vi "ColorScale.vi"(4 "Width":i32=100, 6 "Height":i32=450, 8 "ColorMap":T1=59 items=["Bathymetry9", "BlackBody", "Blue", "BlueBlackRed", "BlueGreenOrange", "BlueHot", "BlueHot256", "BlueRedGreen", "BlueRedGreen256", "BrownViolet", "Classification", "ColdWarm", "Copper", "Cyan", "CyanMagenta", "Cycles", "dBZ14", "dBZ21", "EOSOrangeBlue11", "EOSSpectral11", "Fiddle", "Geo", "Geo32", "Gold", "Grays", "Grays16", "Grays256", "Green", "GreenMagenta16", "LandAndSea", "LandAndSea8", "Magenta", "Mocha", "Mud", "Pastels", "PastelsMap", "PastelsMap20", "PlanetEarth", "PlanetEarth256", "Rainbow", "Rainbow4Cycles", "Rainbow16", "Rainbow256", "RainbowCycle", "Red", "RedWhiteBlue", "RedWhiteBlue256", "RedWhiteGreen", "Relief", "Relief19", "SeaLandAndFire", "Spectrum", "SpectrumBlack", "Terrain", "Terrain256", "VioletOrangeYellow", "Web216", "Yellow", "YellowHot", "YellowHot256"], 9 "Low":i32, 10 "High":i32=260) -> (3 "ColorScale":picture)   [LabVIEW 2014]
uses:
  <vilib>/picture/picture.llb/Draw True-Color Pixmap.vi
  ColorMaps.ctl
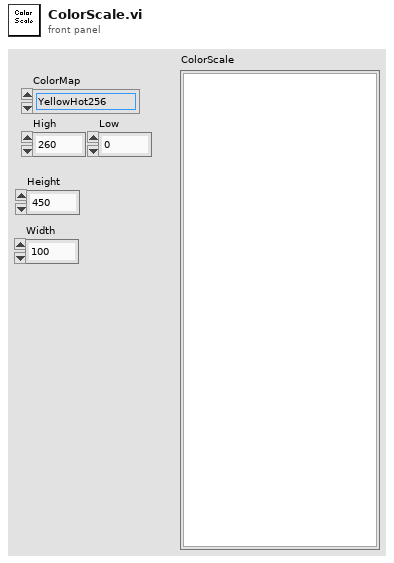
[diagram p1: front panel]
types:
  T1 = typedef "ColorMaps.ctl" = u16
  T2 = cluster{"Width":i16, "Style":enum32{"Solid", "Dash", "Dot", "DashDot", "DashDotDot"}}
  T3 = cluster{"left":i16, "top":i16, "right":i16, "bottom":i16}
  T4 = cluster{"format":enum8{"Decimal", "Scientific", "Engineering", "Binary", "Octal", "Hex"}, "precision":u8}
  T5 = cluster{"horizontal":bool, "left/top":bool, "draw bar":bool, "line color":u32, "text color(black)":u32}
  T6 = cluster{"coordinate 1":i16, "value 1":dbl, "coordinate 2":i16, "value 2":dbl, "log?(F)":bool, "fmt and prec":cluster{"format":enum8{"Decimal", "Scientific", "Engineering", "Binary", "Octal", "Hex"}, "precision":u8}}
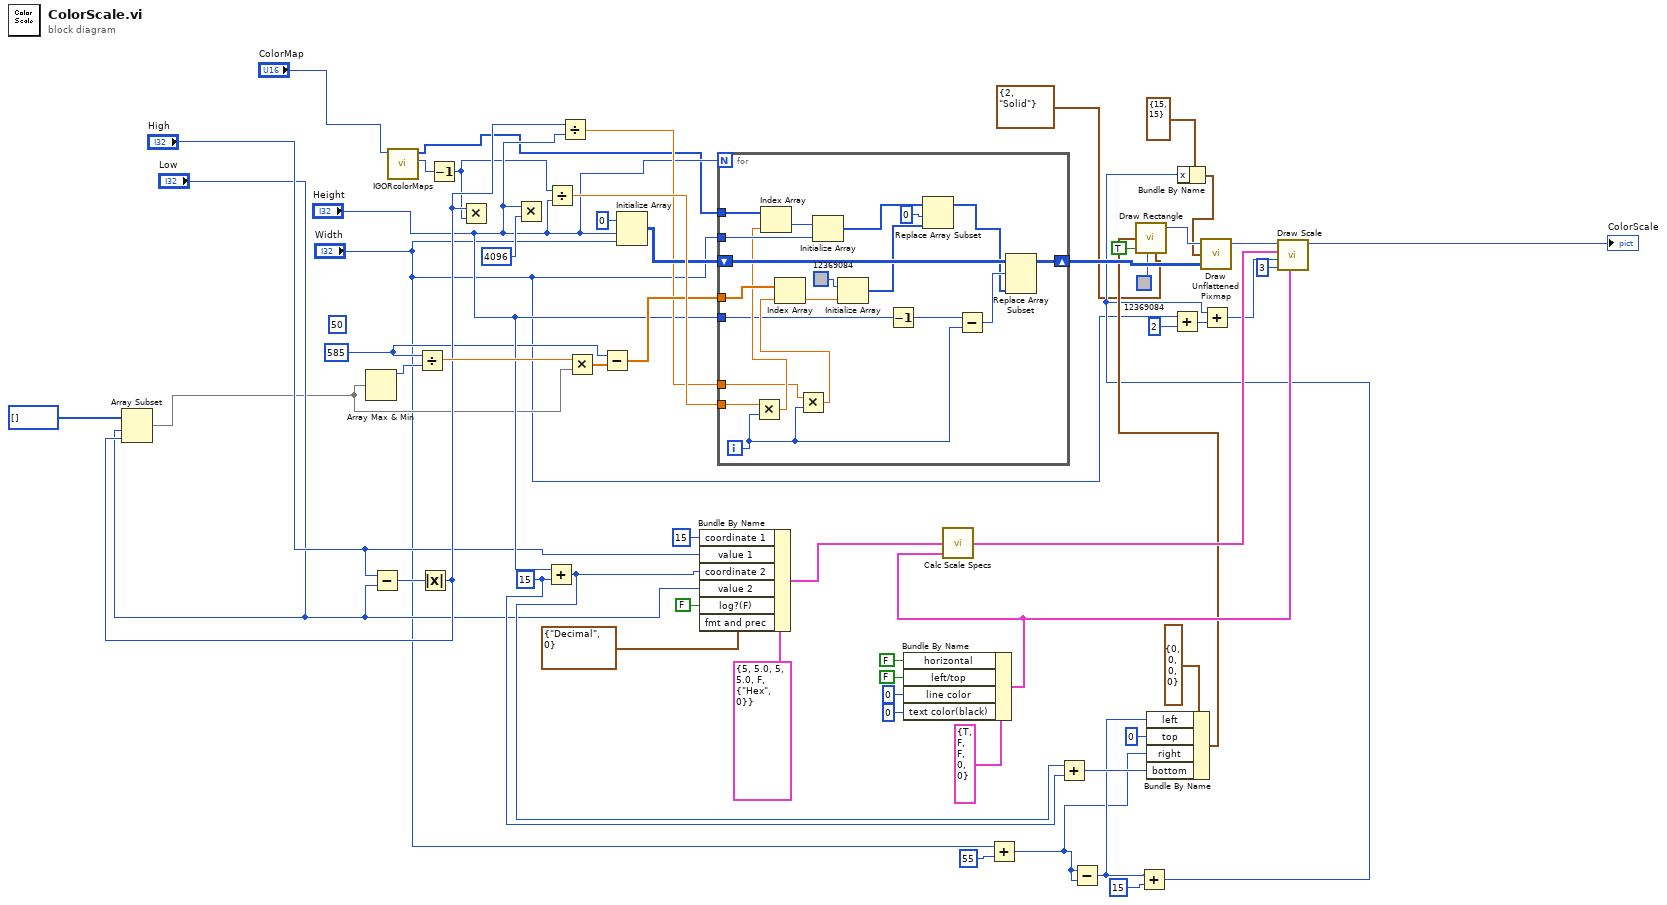
[diagram p0: block diagram]
diagram:
  (unwired) 50
  w3 = 585
  w37 = 15 ("y")
  n1 = Subtract(x="High", y="Low") -> (x-y=w20:i32)
  n2 = call "IGORcolorMaps.vi"("ColorMaps"="ColorMap") -> ("Length"=w9:i32, "ColorMapOut"=w4:u32[])  [unwired: 9 in]
  n3 = Absolute Value(x=w20) -> (abs(x)=w12:i32)
  n4 = Array Subset(array=i32[] [] ("HistOut"), index="Low", length=w12) -> (w5:i32[])
  n5 = Array Max & Min(array=w5) -> (max value=w18:i32)  [unwired: 3 out]
  n6 = Divide(x=w3, y=w18) -> (x/y=w17:dbl)
  n7 = Decrement(x=w9) -> (x-1=w10:i32)
  n8 = Multiply(x=w12, y=w10) -> ()  [unwired: 1 out]
  n9 = Multiply(x="Height", y=4096 ("x")) -> ()  [unwired: 1 out]
  n10 = Add(x="Height", y=w37) -> (x+y=w38:i32)
  n11 = Divide(x=w10, y="Height") -> (x/y=w56:dbl)
  n12 = Divide(x=w12, y="Height") -> (x/y=w14:dbl)
  n13 = Multiply(x=w17, y=w5) -> (x*y=w16:dbl[])
  n14 = Subtract(x=w3, y=w16) -> (x-y=w15:dbl[])
  n15 = Initialize Array(u32 0, "Height", "Width") -> (w55:u32[][])
  n16 = Bundle By Name(cluster=T6 {"coordinate 1"=5, "value 1"=5.0, "coordinate 2"=5, "value 2"=5.0, "log?(F)"=FALSE, "fmt and prec"={"format"=enum."Hex", "precision"=0}} ("scale definition"), "coordinate 1"=i16 15, "value 1"="High", "coordinate 2"=w38, "value 2"="Low", "log?(F)"=FALSE, "fmt and prec"=T4 {"format"=enum."Decimal", "precision"=0}) -> (w52:T6)
  n17 = for {
    N: "Height" -> [_]
    tunnel: w56 -> [w78]
    tunnel: w4 -> [w77]
    shift-right: [w75] -> w34
    shift-left: w55 -> [w76]
    tunnel: "Width" -> [w73]
    tunnel: "Height" -> [w61]
    tunnel: w15 -> [w71]
    tunnel: w14 -> [w68]
    i -> [w69]
    n18 = Multiply(x=w78, y=w69) -> (x*y=w70:dbl)
    n19 = Index Array(array=w77, index=w70) -> (element=w74:u32)
    n20 = Multiply(x=w68, y=w69) -> (x*y=w67:dbl)
    n21 = Index Array(array=w71, index=w67) -> (element=w63:dbl)
    n22 = Initialize Array(w74, w73) -> (w65:u32[])
    n23 = Initialize Array(u32 12369084, w63) -> (w62:u32[])
    n24 = Decrement(x=w61) -> (x-1=w60:i32)
    n25 = Replace Array Subset(array=w65, new element=w62, index=0) -> (w66:u32[])
    n26 = Subtract(x=w60, y=w69) -> (x-y=w72:i32)
    n27 = Replace Array Subset(array=w76, new element=w66, index (row)=w72) -> (w75:u32[][])  [unwired: 1 in]
  }
  n28 = Bundle By Name(cluster=T5 {"horizontal"=TRUE, "left/top"=FALSE, "draw bar"=FALSE, "line color"=0, "text color(black)"=0} ("scale attributes"), "horizontal"=FALSE, "left/top"=FALSE, "line color"=u32 0, "text color(black)"=u32 0) -> (w46:T5)
  n29 = call <vilib>:"Calc Scale Specs.vi"("scale definition"=w52, "scale attributes"=w46) -> ("scale specs"=w48:cluster{"coordinate":i16, "label":string}[])  [unwired: 7 in]
  n30 = Add(x="Width", y=55) -> (x+y=w1:i32)
  n31 = Add(x=w38, y=w37) -> (x+y=w36:i32)
  n32 = Subtract(x=w1, y=w1) -> (x-y=w27:i32)
  n33 = Add(x=w27, y=15) -> (x+y=w24:i32)
  n34 = Bundle By Name(cluster=T3 {"left"=0, "top"=0, "right"=0, "bottom"=0} ("rect"), "left"=w27, "top"=i16 0, "right"=w1, "bottom"=w36) -> (w32:T3)
  n35 = call <vilib>:"Draw Rectangle.vi"("rect"=w32, "fill?(F)"=TRUE, "color(black)"=u32 12369084, "pen"=T2 {"Width"=2, "Style"=enum."Solid"}) -> ("new picture"=w33:picture)  [unwired: 5 in]
  n36 = Add(x="Width", y=2) -> (x+y=w25:i32)
  n37 = Bundle By Name(cluster=cluster{"x":i16, "y":i16} {"x"=15, "y"=15} ("top left point(0, 0)"), "x"=w24) -> (w28:cluster{"x":i16, "y":i16})
  n38 = call-poly <vilib>:"Draw Unflattened Pixmap.vi"("picture"=w33, "top left point(0, 0)"=w28, "data (RGB format)"=w34) -> ("new picture"=w49:picture)  [unwired: 6 in]
  n39 = Add(x=w24, y=w25) -> (x+y=w23:i32)
  n40 = call <vilib>:"Draw Scale.vi"("scale attributes"=w46, "tick length(3)"=i16 3, "constant coordinate"=w23, "scale specs"=w48, "picture"=w49) -> ("new picture"=→"ColorScale":picture)  [unwired: 6 in]
